vi "create new obj.vi"(8 "error in (no error)":errorcluster caption="에러 입력(에러 없음)", 11 "log ref":refnum<vi>) -> (0 "error out":errorcluster caption="에러 출력", 3 "GUI Log Class.lvclass":refnum<class "GUI Log Class.lvclass">)   [LabVIEW 2020, in "GUI Log Class.lvclass"]
uses:
  GUI Log Class.lvclass
  GUI Log Class.lvclass/GUI Log Class.ctl
  Accessors/Write log ref.vi
  Accessors/Write appender queue.vi
  log appender.vi
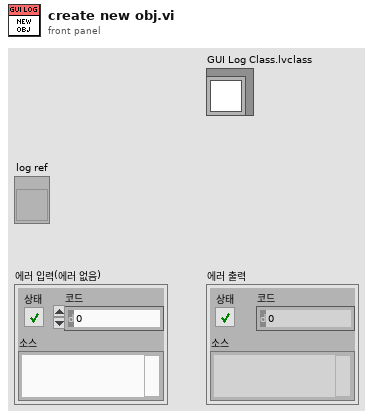
[diagram p1: front panel]
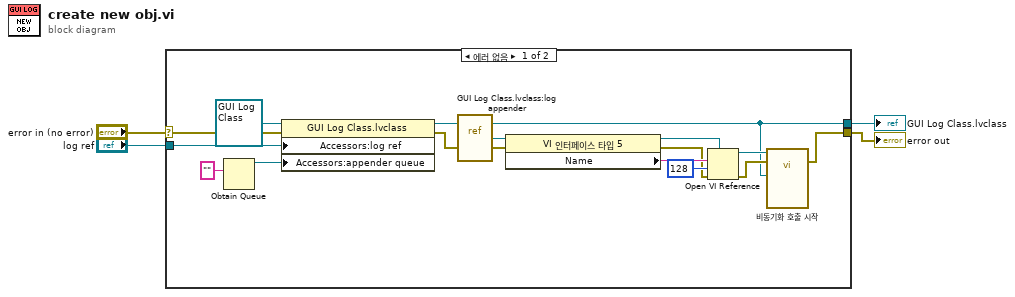
[diagram p0: block diagram]
diagram:
  n1 = case shown="에러 없음" "error in (no error)" {
    selector: "error in (no error)" -> [w18 w20]
    tunnel: [w6 w20] -> w3
    tunnel: [w5 _] -> w2
    tunnel: "log ref" -> [w17 _]
    frame No Error {
      n2 = Obtain Queue(element data type="" ("원소 데이터 타입")) -> (queue out=w15:refnum<queue>)  [unwired: 4 in, 2 out]
      n3 = property class="GUI Log Class.lvclass"(reference=refnum<class "GUI Log Class.lvclass"> refnum ("GUI Log Class.lvclass"), error in=w18, "Accessors:log ref"=w17, "Accessors:appender queue"=w15) -> (reference out=w5:refnum<class "GUI Log Class.lvclass">, error out=w9:errorcluster)
      n4 = vi-ref "GUI Log Class.lvclass:log appender.vi"() -> (w11:refnum<vi>)
      n5 = property class="VI 인터페이스 타입 5"(reference=w11, error in=w9) -> (reference out=w13:refnum<vi>, error out=w8:errorcluster, "Name"=w12:string)
      n6 = Open VI Reference(type specifier VI Refnum (for type only)=w13, vi path=w12, options=128 ("옵션"), error in (no error)=w8) -> (vi reference=w14:refnum<vi>, error out=w7:errorcluster)  [unwired: 2 in]
      n7 = call-by-ref "비동기화 호출 시작"(reference=w14, error in=w7, "GUI Log Class 입력"=w5) -> (error out=w6:errorcluster)  [unwired: 10 in, 2 out]
    }
    frame Error {
    }
  }
  "error out" <- w3
  "GUI Log Class.lvclass" <- w2
